vi "Tapping_Pos.vi"(0 "Orientation":dbl, 1 "Tapping Number":i32) -> (2 "X":dbl, 3 "Y":dbl, 4 "Z":dbl)   [LabVIEW 2011]
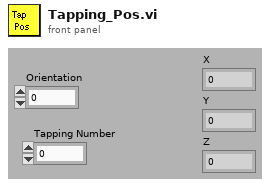
[diagram p1: front panel]
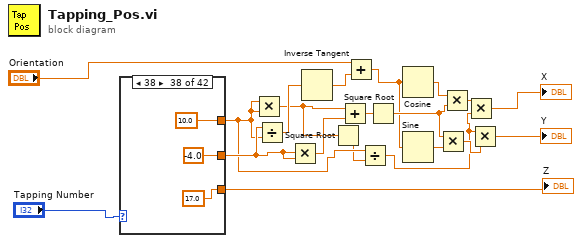
[diagram p0: block diagram]
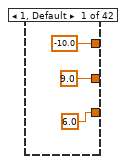
[diagram p2: hidden frame]
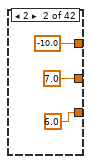
[diagram p3: hidden frame]
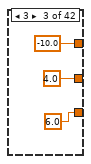
[diagram p4: hidden frame]
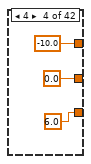
[diagram p5: hidden frame]
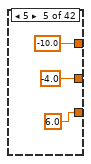
[diagram p6: hidden frame]
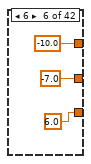
[diagram p7: hidden frame]
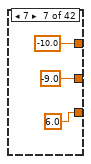
[diagram p8: hidden frame]
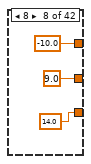
[diagram p9: hidden frame]
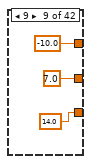
[diagram p10: hidden frame]
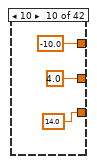
[diagram p11: hidden frame]
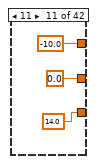
[diagram p12: hidden frame]
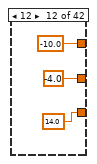
[diagram p13: hidden frame]
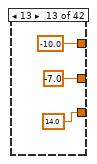
[diagram p14: hidden frame]
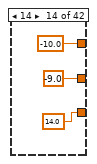
[diagram p15: hidden frame]
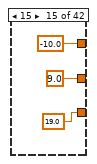
[diagram p16: hidden frame]
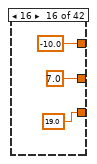
[diagram p17: hidden frame]
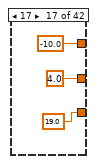
[diagram p18: hidden frame]
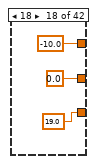
[diagram p19: hidden frame]
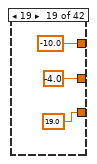
[diagram p20: hidden frame]
diagram:
  n1 = case shown="38" "Tapping Number" {
    tunnel: [-10.0 -10.0 -10.0 -10.0 -10.0 -10.0 -10.0 -10.0 -10.0 -10.0 -10.0 -10.0 -10.0 -10.0 -10.0 -10.0 -10.0 -10.0 -10.0 -10.0 -10.0 10.0 10.0 10.0 10.0 10.0 10.0 10.0 10.0 10.0 10.0 10.0 10.0 10.0 10.0 10.0 10.0 10.0 10.0 10.0 10.0 10.0] -> w9
    tunnel: [9.0 7.0 4.0 0.0 -4.0 -7.0 -9.0 9.0 7.0 4.0 0.0 -4.0 -7.0 -9.0 9.0 7.0 4.0 0.0 -4.0 -7.0 -9.0 -9.0 -7.0 -4.0 0.0 4.0 7.0 9.0 -9.0 -7.0 -4.0 0.0 4.0 7.0 9.0 -9.0 -7.0 -4.0 0.0 4.0 7.0 9.0] -> w13
    tunnel: [6.0 6.0 6.0 6.0 6.0 6.0 6.0 14.0 14.0 14.0 14.0 14.0 14.0 14.0 19.0 19.0 19.0 19.0 19.0 19.0 19.0 2.0 2.0 2.0 2.0 2.0 2.0 2.0 10.0 10.0 10.0 10.0 10.0 10.0 10.0 17.0 17.0 17.0 17.0 17.0 17.0 17.0] -> w14
    frame 1, Default {
    }
    frame 2 {
    }
    frame 3 {
    }
    frame 4 {
    }
    frame 5 {
    }
    frame 6 {
    }
    frame 7 {
    }
    frame 8 {
    }
    frame 9 {
    }
    frame 10 {
    }
    frame 11 {
    }
    frame 12 {
    }
    frame 13 {
    }
    frame 14 {
    }
    frame 15 {
    }
    frame 16 {
    }
    frame 17 {
    }
    frame 18 {
    }
    frame 19 {
    }
    frame 20 {
    }
    frame 21 {
    }
    frame 22 {
    }
    frame 23 {
    }
    frame 24 {
    }
    frame 25 {
    }
    frame 26 {
    }
    frame 27 {
    }
    frame 28 {
    }
    frame 29 {
    }
    frame 30 {
    }
    frame 31 {
    }
    frame 32 {
    }
    frame 33 {
    }
    frame 34 {
    }
    frame 35 {
    }
    frame 36 {
    }
    frame 37 {
    }
    frame 38 {
    }
    frame 39 {
    }
    frame 40 {
    }
    frame 41 {
    }
    frame 42 {
    }
  }
  "Z" <- w14
  n2 = Multiply(x=w9, y=w9) -> (x*y=w8:dbl)
  n3 = Divide(x=w13, y=w9) -> (x/y=w17:dbl)
  n4 = Multiply(x=w13, y=w13) -> (x*y=w15:dbl)
  n5 = Inverse Tangent(1:w17) -> (0:w18:dbl)
  n6 = Square Root(x=w8) -> (sqrt(x)=w7:dbl)
  n7 = Add(x=w8, y=w15) -> (x+y=w16:dbl)
  n8 = Add(x="Orientation", y=w18) -> (x+y=w11:dbl)
  n9 = Divide(x=w9, y=w7) -> (x/y=w4:dbl)
  n10 = Square Root(x=w16) -> (sqrt(x)=w19:dbl)
  n11 = Cosine(x=w11) -> (cos(x)=w12:dbl)
  n12 = Sine(x=w11) -> (sin(x)=w10:dbl)
  n13 = Multiply(x=w19, y=w10) -> (x*y=w5:dbl)
  n14 = Multiply(x=w12, y=w19) -> (x*y=w6:dbl)
  n15 = Multiply(x=w6, y=w4) -> (x*y=→"X":dbl)
  n16 = Multiply(x=w4, y=w5) -> (x*y=→"Y":dbl)
